vi "Mouse click event_demo.vi"() -> ()   [LabVIEW 2012]
panel:
  out "error out":errorcluster
  in  "error in":errorcluster
  in  "Mouse Click":T1(ring)
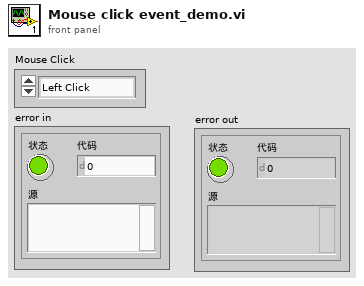
[diagram p1: front panel]
types:
  T1 = enum16{"Left Click", "Left dbClick", "Right Click", "Right dbClick", "Middle Click", "Middle dbClick"}
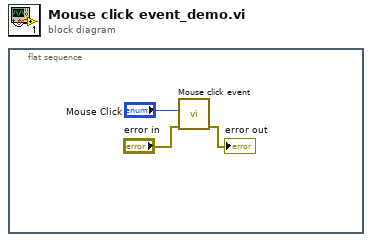
[diagram p0: block diagram]
diagram:
  n1 = flat-sequence {
    frame #0 {
      n2 = call "Mouse click event.vi"("error in"="error in", "Mouse Click"="Mouse Click") -> ("error out"=→"error out":errorcluster)  [unwired: 9 in]
    }
  }
